vi "CreateDataFlowMaps.vi"(8 "error in (no error)":errorcluster, 10 "settling time met":bool, 11 "923x Acquisition Config":T1 {"HighPassFilterState"."Filter State" format="%.2f"; "HighPassFilterState"."IIR Filter Cluster"."Forward Coefficients" format="%.2f"; "HighPassFilterState"."IIR Filter Cluster"."Reverse Coefficients" format="%.2f"; "FixedSizeX32"."InputConfig" items=["AC Coupled", "DC Coupled", "IEPE AC Coupled"]}) -> (0 "error out":errorcluster, 1 "maps":T10[](array[typedef]), 3 "923x Acquisition Config out":T1 {"HighPassFilterState"."Filter State" format="%.2f"; "HighPassFilterState"."IIR Filter Cluster"."Forward Coefficients" format="%.2f"; "HighPassFilterState"."IIR Filter Cluster"."Reverse Coefficients" format="%.2f"; "FixedSizeX32"."InputConfig" items=["AC Coupled", "DC Coupled", "IEPE AC Coupled"]})   [LabVIEW 2017, in "CmsAcquisition.lvlib"]
uses:
  <vilib>/addons/InsightCM/Devices/Shared/Cms/CmsAcquisition/CmsAcquisition.lvlib
  <vilib>/addons/InsightCM/Devices/Shared/Cms/CmsAcquisition/controls/Configuration.ctl
  <vilib>/addons/InsightCM/Devices/Shared/Cms/CmsAcquisition/controls/TachometerConfig.ctl
  <vilib>/addons/InsightCM/Devices/Shared/Cms/CmsAcquisition/controls/FixedSizeArrays.ctl
  <vilib>/LabVIEW Targets/FPGA/cRIO/shared/nicrio_ModuleControls/nicrio_cRIO-9232_ConfigModeRing.ctl
  <vilib>/addons/InsightCM/Devices/Shared/Cms/cRIOWfmAcq/subVIs/RIO Wfm Cust Ctrls/rwfm_SamplingInfo.ctl
  <vilib>/addons/InsightCM/Devices/Shared/Cms/CmsAcquisition/controls/Group.ctl
  <vilib>/addons/InsightCM/Devices/Shared/Cms/CmsAcquisition/controls/Channel.ctl
  <vilib>/addons/InsightCM/Utilities/Analysis/Vibration/controls/HighPassFilterState.ctl
  <vilib>/addons/InsightCM/Devices/Shared/Cms/CmsAcquisition/controls/BurstMode.ctl
  <vilib>/addons/PointValueMap/controls/PointMap.ctl
  <vilib>/addons/PointValueMap/subVIs/Point_Write_double.vi
  <vilib>/addons/PointValueMap/subVIs/Point_Write_i32.vi
  <vilib>/addons/PointValueMap/PointValueMap.lvlib
  <vilib>/addons/InsightCM/Devices/Shared/Cms/cRIOWfmAcq/cRIOWfmLib.lvlib
  <vilib>/addons/InsightCM/Utilities/Analysis/Vibration/VibrationAnalysisFunctions.lvlib
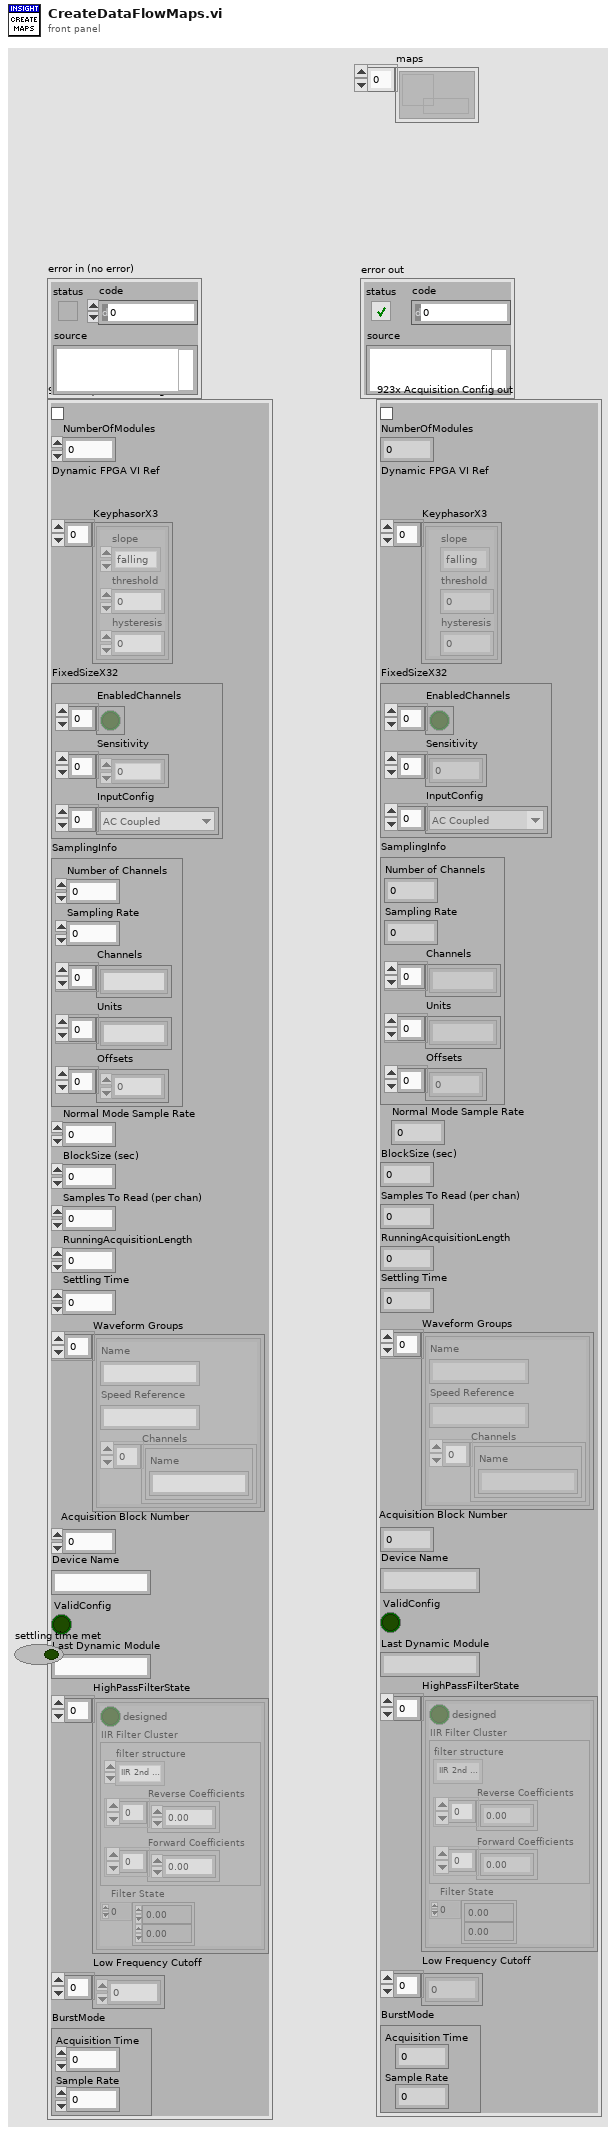
[diagram p1: front panel]
types:
  T1 = typedef "CmsAcquisition.lvlib/Configuration.ctl" = cluster{"Acq":bool, "NumberOfModules":i16, "Dynamic FPGA VI Ref":refnum<k20>, "KeyphasorX3":T2[], "FixedSizeX32":T3, "SamplingInfo":T5, "Normal Mode Sample Rate":dbl, "BlockSize (sec)":dbl, "Samples To Read (per chan)":i32, "RunningAcquisitionLength":dbl, "Settling Time":dbl, "Waveform Groups":T6[], "Acquisition Block Number":i32, "Device Name":string, "ValidConfig":bool, "Last Dynamic Module":string, "HighPassFilterState":T8[], "Low Frequency Cutoff":dbl[], "BurstMode":T9}
  T2 = typedef "CmsAcquisition.lvlib/TachometerConfig.ctl" = cluster{"slope":enum16{"falling", "rising"}, "threshold":dbl, "hysteresis":dbl}
  T3 = typedef "CmsAcquisition.lvlib/FixedSizeArrays.ctl" = cluster{"EnabledChannels":bool[], "Sensitivity":dbl[], "InputConfig":T4[]}
  T4 = typedef "nicrio_cRIO-9232_ConfigModeRing.ctl" = u8
  T5 = typedef "cRIOWfmLib.lvlib/rwfm_SamplingInfo.ctl" = cluster{"Number of Channels":i32, "Sampling Rate":dbl, "Channels":string[], "Units":string[], "Offsets":sgl[]}
  T6 = typedef "CmsAcquisition.lvlib/Group.ctl" = cluster{"Name":string, "Speed Reference":string, "Channels":T7[]}
  T7 = typedef "CmsAcquisition.lvlib/Channel.ctl" = cluster{"Name":string}
  T8 = typedef "VibrationAnalysisFunctions.lvlib/HighPassFilterState.ctl" = cluster{"designed":bool, "IIR Filter Cluster":cluster{"filter structure":enum32{"IIR 2nd Order", "IIR 4th Order"}, "Reverse Coefficients":dbl[], "Forward Coefficients":dbl[]}, "Filter State":dbl[]}
  T9 = typedef "CmsAcquisition.lvlib/BurstMode.ctl" = cluster{"Acquisition Time":dbl, "Sample Rate":dbl}
  T10 = typedef "PointValueMap.lvlib/PointMap.ctl" = refnum<data-value>
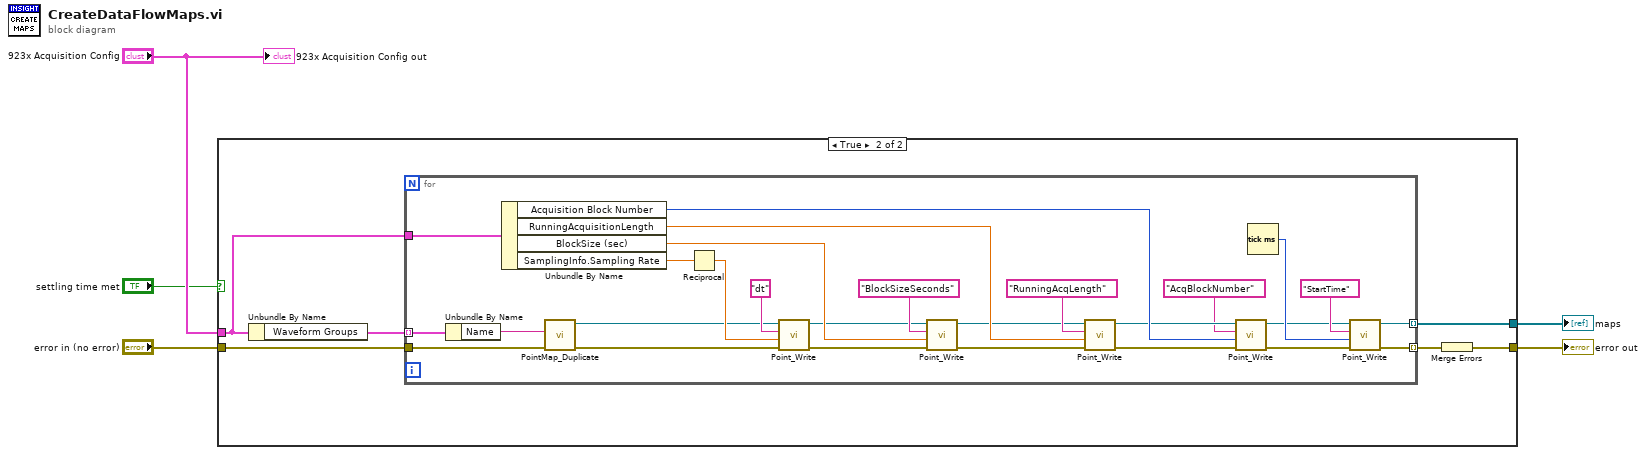
[diagram p0: block diagram]
diagram:
  n1 = case shown="True" "settling time met" {
    tunnel: [w6 w12] -> w5
    tunnel: "error in (no error)" -> [w6 w10]
    tunnel: "923x Acquisition Config" -> [_ w9]
    tunnel: [_ w7] -> w2
    frame False {
    }
    frame True {
      n2 = Unbundle By Name(w9) -> ("Waveform Groups"=w11:T6[])
      n3 = for {
        tunnel: w11 -> [w39] mode=indexing
        tunnel: w10 -> [w37]
        tunnel: w9 -> [w23]
        tunnel: [w16] -> w8 mode=indexing
        tunnel: [w15] -> w7 mode=indexing
        n4 = Unbundle By Name(w39) -> ("Name"=w38:string)
        n5 = Unbundle By Name(w23) -> ("Acquisition Block Number"=w33:i32, "RunningAcquisitionLength"=w34:dbl, "BlockSize (sec)"=w36:dbl, "SamplingInfo.Sampling Rate"=w35:dbl)
        n6 = call <vilib>:"PointMap_Duplicate.vi"("error in (no error)"=w37, "Source Map Name"=w38) -> ("error out"=w21:errorcluster, "Map Out"=w22:T10)  [unwired: 8 in]
        n7 = Reciprocal(x=w35) -> (1/x=w27:dbl)
        n8 = call-poly <vilib>:"Point_Write.vi"("Error In"=w21, "Value"=w27, "Tag"="dt", "Map"=w22) -> ("Error Out"=w29:errorcluster, "Map Out"=w28:T10)  [unwired: 6 in]
        n9 = call-poly <vilib>:"Point_Write.vi"("Error In"=w29, "Value"=w36, "Tag"="BlockSizeSeconds", "Map"=w28) -> ("Error Out"=w13:errorcluster, "Map Out"=w14:T10)  [unwired: 6 in]
        n10 = call-poly <vilib>:"Point_Write.vi"("Error In"=w13, "Value"=w34, "Tag"="RunningAcqLength", "Map"=w14) -> ("Error Out"=w25:errorcluster, "Map Out"=w26:T10)  [unwired: 6 in]
        n11 = call-poly <vilib>:"Point_Write.vi"("Error In"=w25, "Value"=w33, "Tag"="AcqBlockNumber", "Map"=w26) -> ("Error Out"=w17:errorcluster, "Map Out"=w18:T10)  [unwired: 6 in]
        n12 = Tick Count (ms)() -> (millisecond timer value=w19:u32)
        n13 = call-poly <vilib>:"Point_Write.vi"("Error In"=w17, "Value"=w19, "Tag"="StartTime", "Map"=w18) -> ("Error Out"=w16:errorcluster, "Map Out"=w15:T10)  [unwired: 6 in]
      }
      n14 = Merge Errors(w8) -> (w12:errorcluster)
    }
  }
  "error out" <- w5
  "maps" <- w2
  "923x Acquisition Config out" <- "923x Acquisition Config"
